vi "NIP Data.vi"(10 "file path (dialog if empty)":path, 11 "index (row)":i32) -> (1 "file path (dialog if empty) 2":path, 2 "Data":string[][](array[string]))   [LabVIEW 2015]
uses:
  Galobal variable_TI.vi
  <vilib>/Utility/file.llb/Read Delimited Spreadsheet (string).vi
panel:
  out "error out":errorcluster
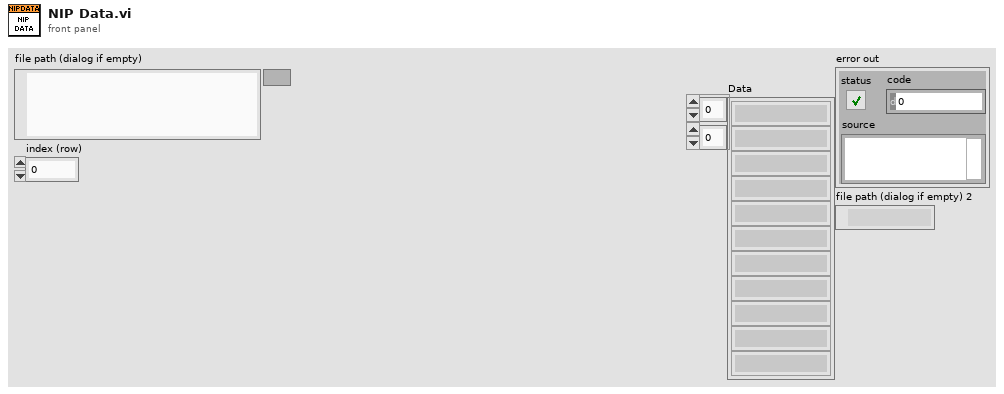
[diagram p1: front panel]
types:
  T1 = cluster{"To-A":timestamp, "From-A":timestamp, "From-B":timestamp, "To-B":timestamp, "From-C 1":timestamp, "To-C 1":timestamp, "From-C 2":timestamp, "To-C 2":timestamp, "Shift":string}
  T2 = cluster{"Stn Name":string, "date":string, "time":string, "Operator id":string, "Shift":string, "Error Code":string, "Fail count":string, "Rework":string, "NA":string, "Tested":string}
  T3 = cluster{"To-A":timestamp, "From-A":timestamp, "From-B":timestamp, "To-B":timestamp, "From-C 1":timestamp, "To-C 1":timestamp, "From-C 2":timestamp, "To-C 2":timestamp}
  T4 = cluster{"No. Fail Coun t":string, "Rework Status Count 0\\1":string, "NA Count Max =3 ":string, "Testesd Count  0/1":string, "Error code":string}
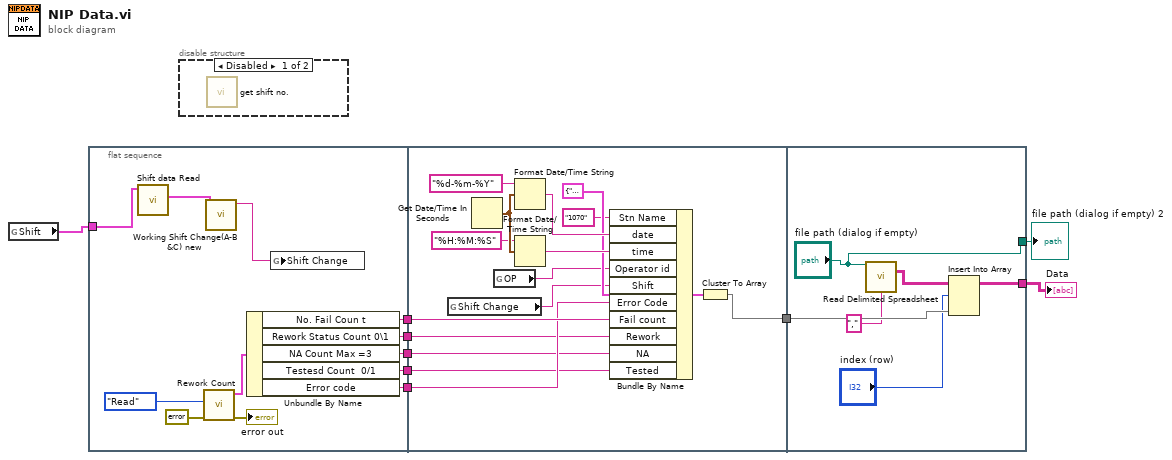
[diagram p0: block diagram]
diagram:
  n1 = global read "Galobal variable_TI.vi" "Shift"() -> (w1:T1)
  n2 = flat-sequence {
    tunnel: [w17] -> w9
    tunnel: [w16] -> w8
    tunnel: [w15] -> w7
    tunnel: [w14] -> w6
    tunnel: [w13] -> w5
    tunnel: w1 -> [w10]
    tunnel: w9 -> [w27]
    tunnel: w8 -> [w26]
    tunnel: w7 -> [w25]
    tunnel: w6 -> [w24]
    tunnel: w5 -> [w23]
    tunnel: [w22] -> w4
    tunnel: w4 -> [w42]
    tunnel: [w40] -> w3
    tunnel: ["file path (dialog if empty)"] -> w2
    frame #0 {
      n3 = call "Shift data Read.vi"("input cluster"=w10) -> ("output cluster"=w12:T3)  [unwired: 10 in]
      n4 = call "Rework Count.vi"("error in"=errorcluster {"status"=FALSE, "code"=0, "source"=""}, "Read /Write"=enum16{"Write", "Read"}."Read") -> ("error out"=→"error out":errorcluster, "data"=w19:T4)  [unwired: 8 in]
      n5 = call "Working Shift Change(A-B &C) new.vi"("input cluster"=w12) -> ("Shift Change"=w11:string)  [unwired: 10 in]
      n6 = Unbundle By Name(w19) -> ("No. Fail Coun t"=w17:string, "Rework Status Count 0\\1"=w15:string, "NA Count Max =3"=w14:string, "Testesd Count  0/1"=w13:string, "Error code"=w16:string)
      n7 = global write "Galobal variable_TI.vi" "Shift Change"(w11) -> ()
    }
    frame #1 {
      n8 = global read "Galobal variable_TI.vi" "Shift Change"() -> (w28:string)
      n9 = Get Date/Time In Seconds() -> (seconds since 1Jan1904=w35:timestamp)
      n10 = global read "Galobal variable_TI.vi" "OP"() -> (w29:string)
      n11 = Format Date/Time String(time format string (%c)="%d-%m-%Y", seconds (now)=w35) -> (date/time string=w36:string)  [unwired: 1 in]
      n12 = Format Date/Time String(time format string (%c)="%H:%M:%S", seconds (now)=w35) -> (date/time string=w33:string)  [unwired: 1 in]
      n13 = Bundle By Name(cluster=T2 {"Stn Name"="", "date"="", "time"="", "Operator id"="", "Shift"="", "Error Code"="", "Fail count"="", "Rework"="", "NA"="", "Tested"=""} ("Write Data"), "Stn Name"="1070", "date"=w36, "time"=w33, "Operator id"=w29, "Shift"=w28, "Error Code"=w26, "Fail count"=w27, "Rework"=w25, "NA"=w24, "Tested"=w23) -> (w32:T2)
      n14 = Cluster To Array(cluster=w32) -> (array=w22:string[])
    }
    frame #2 {
      n15 = call-poly <vilib>:"Read Delimited Spreadsheet.vi"("file path (dialog if empty)"="file path (dialog if empty)", "delimiter (\\t)"="," ("delimiter (\\t)")) -> ("all rows"=w43:string[][])  [unwired: 8 in, 5 out]
      n16 = Insert Into Array(array=w43, index (row)="index (row)", new element=w42) -> (w40:string[][])  [unwired: 1 in]
    }
  }
  n17 = disable-structure shown="Disabled" {
    frame Disabled {
      n18 = call "get shift no..vi"() -> ()  [unwired: 11 in, 1 out]
    }
    frame Enabled {
    }
  }
  "Data" <- w3
  "file path (dialog if empty) 2" <- w2
